vi "Write Header Information.vi"(8 "error in (no error)":errorcluster, 11 "Save Image in":refnum<class "Save Image.lvclass">) -> (0 "error out":errorcluster, 3 "Save Image out":refnum<class "Save Image.lvclass">)   [LabVIEW 2018, in "Save Image.lvclass"]
uses:
  Save Image.lvclass
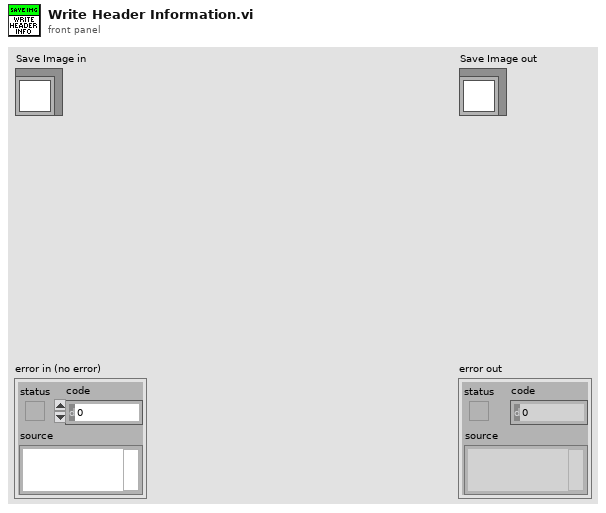
[diagram p1: front panel]
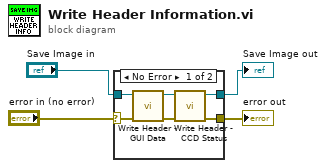
[diagram p0: block diagram]
diagram:
  n1 = case shown="No Error" "error in (no error)" {
    selector: "error in (no error)" -> [w9 w11]
    tunnel: [w5 w11] -> w3
    tunnel: [w6 w12] -> w1
    tunnel: "Save Image in" -> [w10 w12]
    frame No Error {
      n2 = call "Write Header - GUI Data.vi"("error in (no error)"=w9, "Save Image in"=w10) -> ("error out"=w8:errorcluster, "Save Image out"=w7:refnum<class "Save Image.lvclass">)  [unwired: 8 in]
      n3 = call "Write Header - CCD Status.vi"("error in (no error)"=w8, "Save Image in"=w7) -> ("error out"=w5:errorcluster, "Save Image out"=w6:refnum<class "Save Image.lvclass">)  [unwired: 8 in]
    }
    frame Error {
    }
  }
  "error out" <- w3
  "Save Image out" <- w1
